vi "Periodic Tasks.vi"(8 "error in":errorcluster) -> ()   [LabVIEW 2018]
doc: "This VI runs in parallel to other tasks. It can contain as many user-defined periodic loops as you need. These can carry out PID or other sorts of timed response."
uses:
  <vilib>/Rock Robotics/WPI/Solenoid/WPI_SolenoidValue.ctl
  <vilib>/Rock Robotics/WPI/Utilities/WPI_GetSetVariantRefNum.vi
  <vilib>/Rock Robotics/WPI/Solenoid/WPI_SolenoidSetEnum.vi
  Robot Global Data.vi
  <vilib>/Rock Robotics/WPI/RobotDrive/WPI_RobotDriveArcadeDrive_Standard(NoSaturation).vi
  <vilib>/Rock Robotics/Network Tables/NT Write Numeric Array.vi
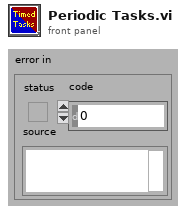
[diagram p1: front panel]
types:
  T1 = typedef "WPI_JoystickDevRef.ctl" = cluster{"Device":T2}
  T2 = typedef "WPI_JoystickDeviceEnum.ctl" = enum16{"USB 0", "USB 1", "USB 2", "USB 3", "USB 4", "USB 5"}
  T3 = typedef "WPI_SolenoidDevRef.ctl" = cluster{"DevStatus":errorcluster, "Pneumatics Control Module":u8, "Forward Solenoid Channel":T4, "Reverse Solenoid Channel":T4}
  T4 = typedef "WPI_SolenoidChannel.ctl" = enum8{"Solenoid 0", "Solenoid 1", "Solenoid 2", "Solenoid 3", "Solenoid 4", "Solenoid 5", "Solenoid 6", "Solenoid 7", "Invalid"}
  T5 = typedef "WPI_AccelerometerDevRef.ctl" = cluster{"DevStatus":errorcluster, "Scaling":T6, "Analog Channels":T7, "I2C Bus":T9, "SPI Bus":T10, "Accel Range":T11, "ADXL Axes":T12, "Handle":i32, "Device Address":u8, "Accel Type":enum16{"Analog", "ADXL345 I2C", "ADXL345 SPI", "Internal", "ADXL362 SPI"}}
  T6 = typedef "WPI_AccelerometerScaling.ctl" = cluster{"Gain (VoltsPerG)":dbl, "Center Voltage":dbl}
  T7 = typedef "WPI_AccelerometerAnalogChannels.ctl" = cluster{"X-Axis":T8, "Y-Axis":T8, "Z-Axis":T8}
  T8 = typedef "FPGA_AIChannel.ctl" = enum8{"AI 0", "AI 1", "AI 2", "AI 3", "AI MXP 0", "AI MXP 1", "AI MXP 2", "AI MXP 3", "Invalid"}
  T9 = typedef "i2c_bus.ctl" = enum16{"I2C On-Board", "I2C MXP", "Invalid"}
  T10 = typedef "spi_bus.ctl" = enum16{"SPI On-Board, CS0", "SPI On-Board, CS1", "SPI On-Board, CS2", "SPI On-Board, CS3", "SPI MXP", "Invalid"}
  T11 = typedef "ADXL345 Range.ctl" = u8
  T12 = typedef "WPI_AccelerometerADXL345 Axes.ctl" = cluster{"X-Axis":bool, "Y-Axis":bool, "Z-Axis":bool}
  T13 = typedef "WPI_SolenoidValue.ctl" = enum16{"Off", "On", "Forward", "Reverse"}
  T14 = typedef "WPI_RobotDriveDevRef.ctl" = cluster{"DevStatus":errorcluster, "Motors[]":T15[], "Square Inputs":bool, "Max Output":dbl}
  T15 = typedef "WPI_MotorControlDeviceRef.ctl" = cluster{"DeviceStatus":errorcluster, "Type":T16, "PWM":cluster{"PWM Channel":T17, "DeadBand":T18}, "CAN":cluster{"Device Number":u8, "SetOutput VI Ref":variant, "GetOutput VI Ref":variant, "Enable VI Ref":variant, "Disable VI Ref":variant, "Data":variant}, "Invert":bool, "DIO PWM":cluster{"PWM \"Enable\" Channel":T17, "DIOChannel":T19, "PWM Rate":dbl}}
  T16 = typedef "WPI_MotorControlType.ctl" = enum16{"PWM", "CAN", "DIO PWM"}
  T17 = typedef "FPGA_DIOPWMChannel.ctl" = enum8{"PWM 0", "PWM 1", "PWM 2", "PWM 3", "PWM 4", "PWM 5", "PWM 6", "PWM 7", "PWM 8", "PWM 9", "PWM MXP 0", "PWM MXP 1", "PWM MXP 2", "PWM MXP 3", "PWM MXP 4", "PWM MXP 5", "PWM MXP 6", "PWM MXP 7", "PWM MXP 8", "PWM MXP 9", "Invalid"}
  T18 = typedef "WPI_PWMDeadband.ctl" = cluster{"Name":string, "maxPositivePwm":i32, "minPositivePwm":i32, "centerPwm":i32, "maxNegativePwm":i32, "minNegativePwm":i32, "angularRange":u16}
  T19 = typedef "FPGA_DIOChannel.ctl" = enum8{"DIO 0", "DIO 1", "DIO 2", "DIO 3", "DIO 4", "DIO 5", "DIO 6", "DIO 7", "DIO 8", "DIO 9", "DIO MXP 0", "DIO MXP 1", "DIO MXP 2", "DIO MXP 3", "DIO MXP 4", "DIO MXP 5", "DIO MXP 6", "DIO MXP 7", "DIO MXP 8", "DIO MXP 9", "DIO MXP 10", "DIO MXP 11", "DIO MXP 12", "DIO MXP 13", "DIO MXP 14", "DIO MXP 15", "SPI Port CS1", "SPI Port CS2", "SPI Port CS3", "SPI Port MISO", "SPI Port MOSI", "Invalid"}
  T20 = cluster{"X-Axis":dbl, "Y-Axis":dbl, "Z-Axis":dbl}
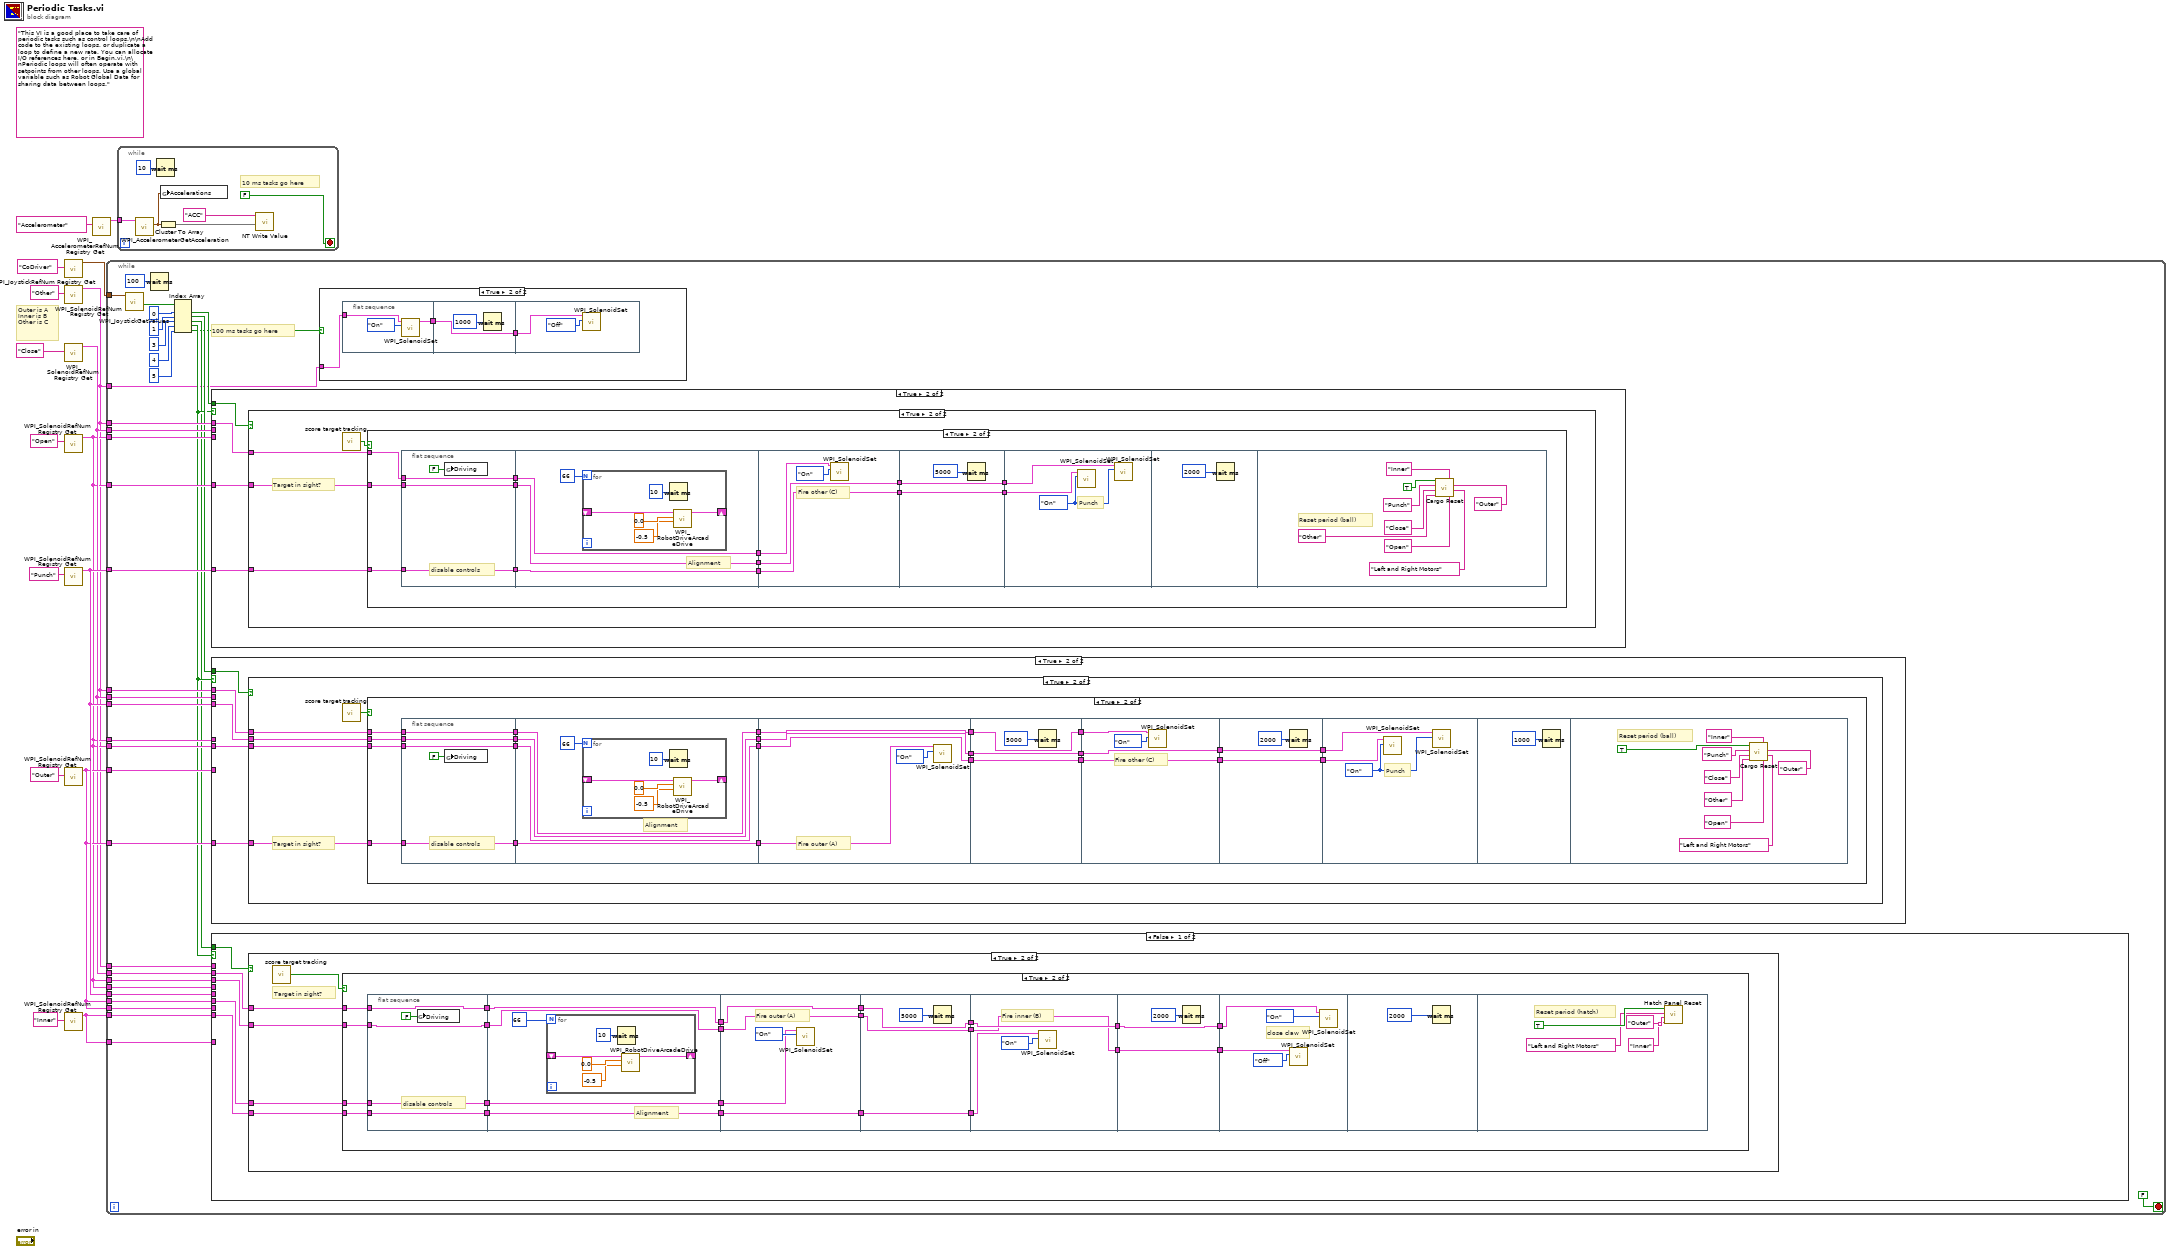
[diagram p0: block diagram]
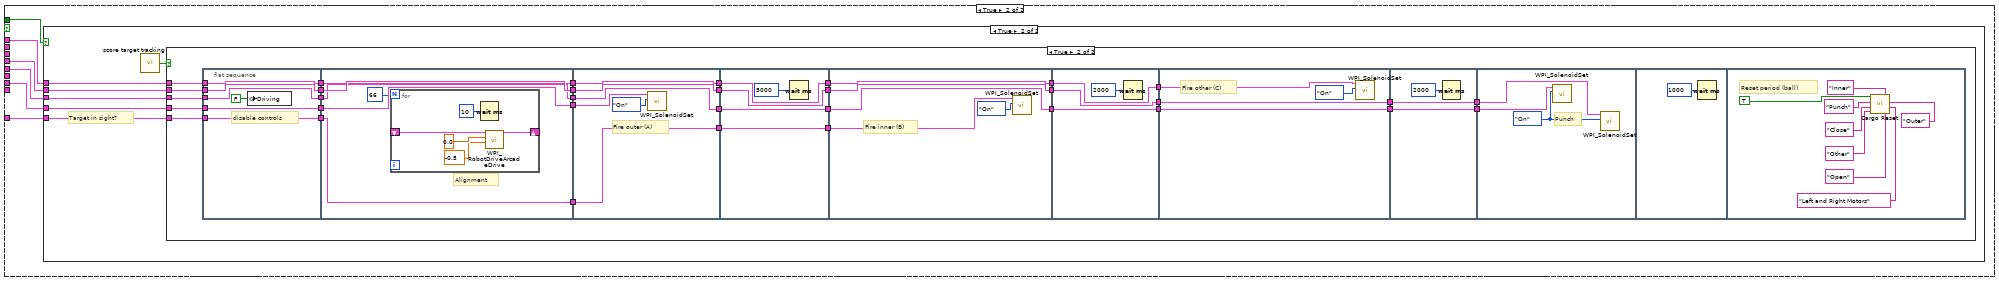
[diagram p5: hidden frame]
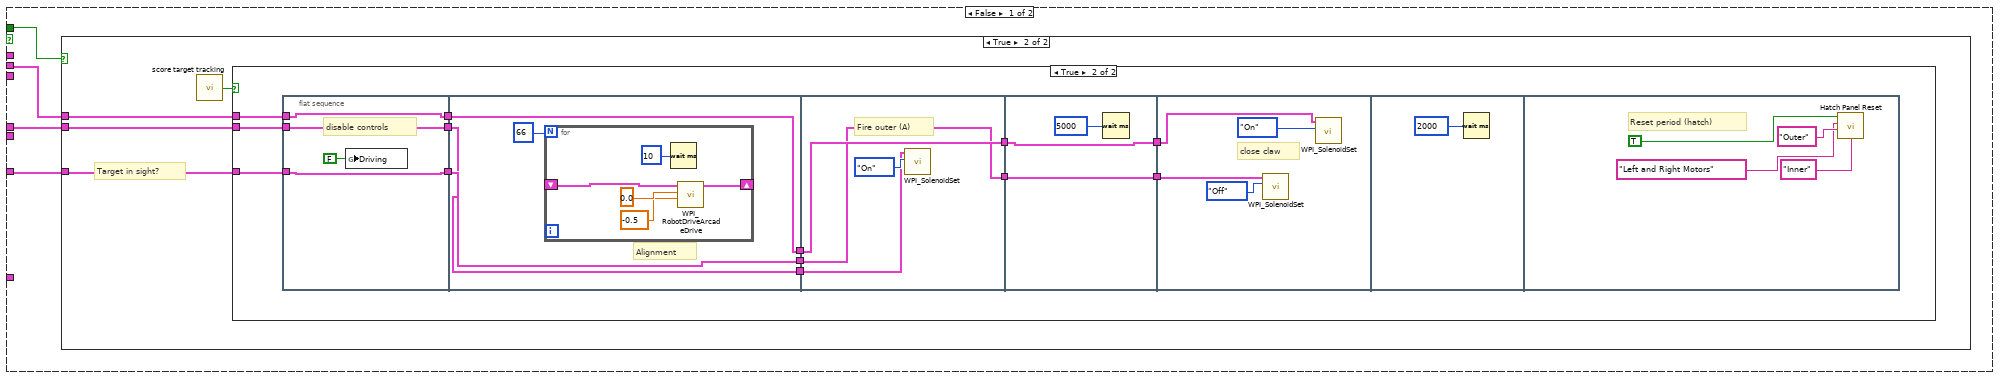
[diagram p8: hidden frame]
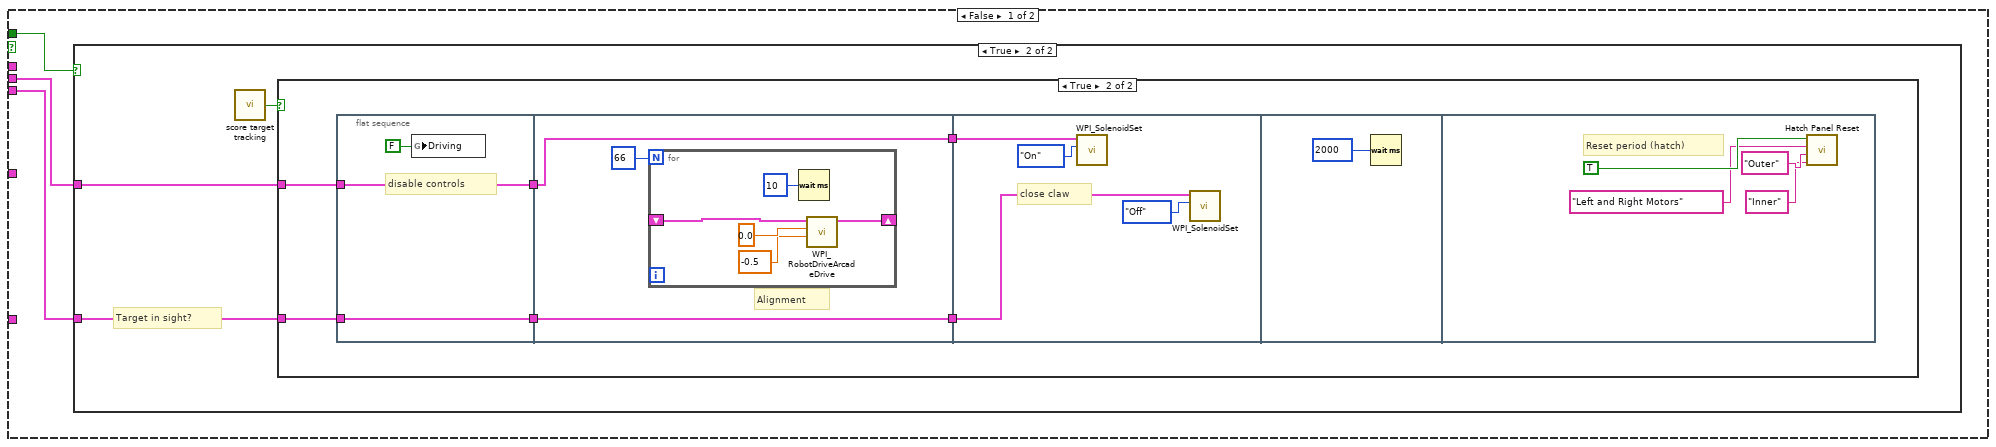
[diagram p13: hidden frame]
diagram:
  (unwired) "This VI is a good place to take care of periodic tasks such as control loops.\n\nAdd code to the existing loops, or duplicate a loop to define a new rate. You can allocate I/O references here, or in Begin.vi.\n\nPeriodic loops will often operate with setpoints from other loops. Use a global variable such as Robot Global Data for sharing data between loops."
  # "Outer is A\nInner is B\nOther is C"
  n1 = call <vilib>:"WPI_JoystickRefNum Registry Get.vi"("refnum name"="CoDriver") -> ("JoystickDevRef"=w12:T1)  [unwired: 9 in, 1 out]
  n2 = call <vilib>:"WPI_SolenoidRefNum Registry Get.vi"("refnum name"="Other") -> ("SolenoidDevRef"=w3:T3)  [unwired: 9 in, 1 out]
  n3 = call <vilib>:"WPI_SolenoidRefNum Registry Get.vi"("refnum name"="Close") -> ("SolenoidDevRef"=w5:T3)  [unwired: 9 in, 1 out]
  n4 = call <vilib>:"WPI_SolenoidRefNum Registry Get.vi"("refnum name"="Open") -> ("SolenoidDevRef"=w4:T3)  [unwired: 9 in, 1 out]
  n5 = call <vilib>:"WPI_SolenoidRefNum Registry Get.vi"("refnum name"="Punch") -> ("SolenoidDevRef"=w8:T3)  [unwired: 9 in, 1 out]
  n6 = call <vilib>:"WPI_SolenoidRefNum Registry Get.vi"("refnum name"="Outer") -> ("SolenoidDevRef"=w7:T3)  [unwired: 9 in, 1 out]
  n7 = call <vilib>:"WPI_SolenoidRefNum Registry Get.vi"("refnum name"="Inner") -> ("SolenoidDevRef"=w6:T3)  [unwired: 9 in, 1 out]
  n8 = call <vilib>:"WPI_AccelerometerRefNum Registry Get.vi"("refnum name"="Accelerometer") -> ("AccelerometerDevRef"=w2:T5)  [unwired: 9 in, 1 out]
  n9 = while {
    tunnel: w12 -> [w50]
    tunnel: w3 -> [w44]
    tunnel: w4 -> [w43]
    tunnel: w8 -> [w42]
    tunnel: w5 -> [w40]
    tunnel: w4 -> [w39]
    tunnel: w8 -> [w38]
    tunnel: w4 -> [w37]
    tunnel: w7 -> [w36]
    tunnel: w3 -> [w35]
    tunnel: w7 -> [w33]
    tunnel: w5 -> [w32]
    tunnel: w4 -> [w31]
    tunnel: w4 -> [w29]
    tunnel: w8 -> [w28]
    tunnel: w7 -> [w27]
    tunnel: w6 -> [w26]
    tunnel: w3 -> [w25]
    tunnel: w7 -> [w24]
    tunnel: w6 -> [w23]
    tunnel: w5 -> [w22]
    tunnel: w4 -> [w21]
    tunnel: w3 -> [w17]
    stop <- FALSE stop-if-true
    # "100 ms tasks go here"
    n10 = call <vilib>:"WPI_JoystickGetValues.vi"("JoystickDevRef"=w50) -> ("Buttons"=w49:bool[])  [unwired: 6 in, 4 out]
    n11 = Wait (ms)(milliseconds to wait=u32 100) -> ()  [unwired: 1 out]
    n12 = Index Array(array=w49, index #1=0, index #2=1, index #3=3, index #4=4, index #5=5) -> (element #1=w41:bool, element #2=w34:bool, element #3=w20:bool, element #4=w30:bool, element #5=w18:bool)
    n13 = case shown="True" w30 {
      tunnel: w44 -> [_ w396]
      tunnel: w43 -> [_ w395]
      tunnel: w42 -> [_ w394]
      tunnel: w41 -> [w363 w393]
      tunnel: w40 -> [w362 _]
      tunnel: w39 -> [w361 _]
      frame False {
        n14 = case shown="True" w363 {
          tunnel: w362 -> [_ w366]
          tunnel: w361 -> [_ w365]
          frame False {
          }
          frame True {
            # "Target in sight?"
            n15 = call "score target tracking.vi"() -> ("Boolean"=w364:bool)
            n16 = case shown="True" w364 {
              tunnel: w366 -> [_ w372]
              tunnel: w365 -> [_ w371]
              frame False {
              }
              frame True {
                n17 = flat-sequence {
                  tunnel: [w375] -> w370
                  tunnel: w372 -> [w375]
                  tunnel: [w374] -> w368
                  tunnel: w371 -> [w374]
                  tunnel: w370 -> [w378]
                  tunnel: [w378] -> w369
                  tunnel: w368 -> [w377]
                  tunnel: [w377] -> w367
                  tunnel: w369 -> [w387]
                  tunnel: w367 -> [w384]
                  frame #0 {
                    # "disable controls"
                    n18 = global write "Robot Global Data.vi" "Driving"(FALSE) -> ()
                  }
                  frame #1 {
                    # "Alignment"
                    n19 = for {
                      N: 66 -> [_]
                      shift-right: [w383] -> _
                      shift-left: _ -> [w382]
                      n20 = Wait (ms)(milliseconds to wait=u32 10) -> ()  [unwired: 1 out]
                      n21 = call-poly <vilib>:"WPI_RobotDriveArcadeDrive.vi"("Y axis value"=-0.5, "X axis value"=0.0, "RobotDriveDevRef"=w382) -> ("RobotDriveDevRef"=w383:T14)  [unwired: 6 in, 2 out]
                    }
                  }
                  frame #2 {
                    # "close claw"
                    n22 = call-poly <vilib>:"WPI_SolenoidSet.vi"("Value"=WPI_SolenoidValue."On", "SolenoidDevRef"=w387) -> ()  [unwired: 8 in, 2 out]
                    n23 = call-poly <vilib>:"WPI_SolenoidSet.vi"("Value"=WPI_SolenoidValue."Off", "SolenoidDevRef"=w384) -> ()  [unwired: 8 in, 2 out]
                  }
                  frame #3 {
                    n24 = Wait (ms)(milliseconds to wait=u32 2000) -> ()  [unwired: 1 out]
                  }
                  frame #4 {
                    # "Reset period (hatch)"
                    n25 = call "Hatch Panel Reset.vi"("InnerRefnum"="Inner", "OuterRefnum"="Outer", "DriveRefnum"="Left and Right Motors", "HatchReset?"=TRUE) -> ()
                  }
                }
              }
            }
          }
        }
      }
      frame True {
        n26 = case shown="True" w393 {
          tunnel: w396 -> [_ w400]
          tunnel: w395 -> [_ w399]
          tunnel: w394 -> [_ w398]
          frame False {
          }
          frame True {
            # "Target in sight?"
            n27 = call "score target tracking.vi"() -> ("Boolean"=w397:bool)
            n28 = case shown="True" w397 {
              tunnel: w400 -> [_ w409]
              tunnel: w399 -> [_ w408]
              tunnel: w398 -> [_ w407]
              frame False {
              }
              frame True {
                n29 = flat-sequence {
                  tunnel: [w417] -> w406
                  tunnel: [w416] -> w404
                  tunnel: [w415] -> w402
                  tunnel: w407 -> [w415]
                  tunnel: w408 -> [w416]
                  tunnel: w409 -> [w417]
                  tunnel: w406 -> [w421]
                  tunnel: [w421] -> w405
                  tunnel: w404 -> [w420]
                  tunnel: [w420] -> w403
                  tunnel: w402 -> [w419]
                  tunnel: [w419] -> w401
                  tunnel: w405 -> [w430]
                  tunnel: [w428] -> w413
                  tunnel: w403 -> [w428]
                  tunnel: [w427] -> w412
                  tunnel: w401 -> [w427]
                  tunnel: w413 -> [w433]
                  tunnel: [w433] -> w411
                  tunnel: w412 -> [w432]
                  tunnel: [w432] -> w410
                  tunnel: w411 -> [w436]
                  tunnel: w410 -> [w435]
                  frame #0 {
                    # "disable controls"
                    n30 = global write "Robot Global Data.vi" "Driving"(FALSE) -> ()
                  }
                  frame #1 {
                    # "Alignment"
                    n31 = for {
                      N: 66 -> [_]
                      shift-right: [w426] -> _
                      shift-left: _ -> [w425]
                      n32 = Wait (ms)(milliseconds to wait=u32 10) -> ()  [unwired: 1 out]
                      n33 = call-poly <vilib>:"WPI_RobotDriveArcadeDrive.vi"("Y axis value"=-0.5, "X axis value"=0.0, "RobotDriveDevRef"=w425) -> ("RobotDriveDevRef"=w426:T14)  [unwired: 6 in, 2 out]
                    }
                  }
                  frame #2 {
                    # "Fire other (C)"
                    n34 = call-poly <vilib>:"WPI_SolenoidSet.vi"("Value"=WPI_SolenoidValue."On", "SolenoidDevRef"=w430) -> ()  [unwired: 8 in, 2 out]
                  }
                  frame #3 {
                    n35 = Wait (ms)(milliseconds to wait=u32 5000) -> ()  [unwired: 1 out]
                  }
                  frame #4 {
                    w434 = WPI_SolenoidValue."On" ("Value")
                    # "Punch"
                    n36 = call-poly <vilib>:"WPI_SolenoidSet.vi"("Value"=w434, "SolenoidDevRef"=w435) -> ()  [unwired: 8 in, 2 out]
                    n37 = call-poly <vilib>:"WPI_SolenoidSet.vi"("Value"=w434, "SolenoidDevRef"=w436) -> ()  [unwired: 8 in, 2 out]
                  }
                  frame #5 {
                    n38 = Wait (ms)(milliseconds to wait=u32 2000) -> ()  [unwired: 1 out]
                  }
                  frame #6 {
                    # "Reset period (ball)"
                    n39 = call "Cargo Reset.vi"("Open Refnum"="Open" ("refnum name"), "Drive Refnum"="Left and Right Motors" ("DriveRefnum"), "Outer Refnum"="Outer" ("OuterRefnum"), "Inner Refnum"="Inner" ("InnerRefnum"), "Other Refnum"="Other" ("refnum name"), "Close Refnum"="Close" ("refnum name"), "Punch Refnum"="Punch" ("refnum name"), "Ball reset?"=TRUE) -> ()
                  }
                }
              }
            }
          }
        }
      }
    }
    n40 = case shown="True" w30 {
      tunnel: w38 -> [_ w290]
      tunnel: w37 -> [_ w289]
      tunnel: w36 -> [_ w288]
      tunnel: w35 -> [_ w287]
      tunnel: w34 -> [w239 w286]
      tunnel: w33 -> [w238 _]
      tunnel: w32 -> [w237 _]
      tunnel: w31 -> [w236 _]
      frame False {
        n41 = case shown="True" w239 {
          tunnel: w238 -> [_ w243]
          tunnel: w237 -> [_ w242]
          tunnel: w236 -> [_ w241]
          frame False {
          }
          frame True {
            # "Target in sight?"
            n42 = call "score target tracking.vi"() -> ("Boolean"=w240:bool)
            n43 = case shown="True" w240 {
              tunnel: w243 -> [_ w252]
              tunnel: w242 -> [_ w251]
              tunnel: w241 -> [_ w250]
              frame False {
              }
              frame True {
                n44 = flat-sequence {
                  tunnel: [w260] -> w249
                  tunnel: w252 -> [w260]
                  tunnel: [w259] -> w247
                  tunnel: w251 -> [w259]
                  tunnel: [w258] -> w245
                  tunnel: w250 -> [w258]
                  tunnel: w249 -> [w264]
                  tunnel: [w264] -> w248
                  tunnel: w247 -> [w263]
                  tunnel: [w263] -> w246
                  tunnel: w245 -> [w262]
                  tunnel: [w262] -> w244
                  tunnel: w248 -> [w272]
                  tunnel: [w271] -> w256
                  tunnel: w246 -> [w271]
                  tunnel: [w270] -> w255
                  tunnel: w244 -> [w270]
                  tunnel: w256 -> [w276]
                  tunnel: [w276] -> w254
                  tunnel: w255 -> [w275]
                  tunnel: [w275] -> w253
                  tunnel: w254 -> [w280]
                  tunnel: w253 -> [w277]
                  frame #0 {
                    # "disable controls"
                    n45 = global write "Robot Global Data.vi" "Driving"(FALSE) -> ()
                  }
                  frame #1 {
                    # "Alignment"
                    n46 = for {
                      N: 66 -> [_]
                      shift-right: [w269] -> _
                      shift-left: _ -> [w268]
                      n47 = Wait (ms)(milliseconds to wait=u32 10) -> ()  [unwired: 1 out]
                      n48 = call-poly <vilib>:"WPI_RobotDriveArcadeDrive.vi"("Y axis value"=-0.5, "X axis value"=0.0, "RobotDriveDevRef"=w268) -> ("RobotDriveDevRef"=w269:T14)  [unwired: 6 in, 2 out]
                    }
                  }
                  frame #2 {
                    # "Fire outer (A)"
                    n49 = call-poly <vilib>:"WPI_SolenoidSet.vi"("Value"=WPI_SolenoidValue."On", "SolenoidDevRef"=w272) -> ()  [unwired: 8 in, 2 out]
                  }
                  frame #3 {
                    n50 = Wait (ms)(milliseconds to wait=u32 5000) -> ()  [unwired: 1 out]
                  }
                  frame #4 {
                    # "close claw"
                    n51 = call-poly <vilib>:"WPI_SolenoidSet.vi"("Value"=WPI_SolenoidValue."Off", "SolenoidDevRef"=w277) -> ()  [unwired: 8 in, 2 out]
                    n52 = call-poly <vilib>:"WPI_SolenoidSet.vi"("Value"=WPI_SolenoidValue."On", "SolenoidDevRef"=w280) -> ()  [unwired: 8 in, 2 out]
                  }
                  frame #5 {
                    n53 = Wait (ms)(milliseconds to wait=u32 2000) -> ()  [unwired: 1 out]
                  }
                  frame #6 {
                    # "Reset period (hatch)"
                    n54 = call "Hatch Panel Reset.vi"("InnerRefnum"="Inner", "OuterRefnum"="Outer", "DriveRefnum"="Left and Right Motors", "HatchReset?"=TRUE) -> ()
                  }
                }
              }
            }
          }
        }
      }
      frame True {
        n55 = case shown="True" w286 {
          tunnel: w290 -> [_ w295]
          tunnel: w289 -> [_ w294]
          tunnel: w288 -> [_ w293]
          tunnel: w287 -> [_ w292]
          frame False {
          }
          frame True {
            # "Target in sight?"
            n56 = call "score target tracking.vi"() -> ("Boolean"=w291:bool)
            n57 = case shown="True" w291 {
              tunnel: w295 -> [_ w307]
              tunnel: w294 -> [_ w306]
              tunnel: w293 -> [_ w305]
              tunnel: w292 -> [_ w304]
              frame False {
              }
              frame True {
                n58 = flat-sequence {
                  tunnel: [w322] -> w303
                  tunnel: w307 -> [w322]
                  tunnel: [w321] -> w301
                  tunnel: w306 -> [w321]
                  tunnel: [w320] -> w299
                  tunnel: w305 -> [w320]
                  tunnel: [w319] -> w297
                  tunnel: w304 -> [w319]
                  tunnel: w303 -> [w327]
                  tunnel: [w327] -> w302
                  tunnel: w301 -> [w326]
                  tunnel: [w326] -> w300
                  tunnel: w299 -> [w325]
                  tunnel: [w325] -> w298
                  tunnel: w297 -> [w324]
                  tunnel: [w324] -> w296
                  tunnel: [w337] -> w317
                  tunnel: w302 -> [w337]
                  tunnel: [w336] -> w316
                  tunnel: w300 -> [w336]
                  tunnel: w298 -> [w334]
                  tunnel: [w333] -> w315
                  tunnel: w296 -> [w333]
                  tunnel: w317 -> [w341]
                  tunnel: [w341] -> w314
                  tunnel: w316 -> [w340]
                  tunnel: [w340] -> w313
                  tunnel: w315 -> [w339]
                  tunnel: [w339] -> w312
                  tunnel: [w345] -> w311
                  tunnel: w314 -> [w345]
                  tunnel: [w344] -> w310
                  tunnel: w313 -> [w344]
                  tunnel: w312 -> [w342]
                  tunnel: w311 -> [w348]
                  tunnel: [w348] -> w309
                  tunnel: w310 -> [w347]
                  tunnel: [w347] -> w308
                  tunnel: w309 -> [w351]
                  tunnel: w308 -> [w350]
                  frame #0 {
                    # "disable controls"
                    n59 = global write "Robot Global Data.vi" "Driving"(FALSE) -> ()
                  }
                  frame #1 {
                    # "Alignment"
                    n60 = for {
                      N: 66 -> [_]
                      shift-right: [w332] -> _
                      shift-left: _ -> [w331]
                      n61 = Wait (ms)(milliseconds to wait=u32 10) -> ()  [unwired: 1 out]
                      n62 = call-poly <vilib>:"WPI_RobotDriveArcadeDrive.vi"("Y axis value"=-0.5, "X axis value"=0.0, "RobotDriveDevRef"=w331) -> ("RobotDriveDevRef"=w332:T14)  [unwired: 6 in, 2 out]
                    }
                  }
                  frame #2 {
                    # "Fire outer (A)"
                    n63 = call-poly <vilib>:"WPI_SolenoidSet.vi"("Value"=WPI_SolenoidValue."On", "SolenoidDevRef"=w334) -> ()  [unwired: 8 in, 2 out]
                  }
                  frame #3 {
                    n64 = Wait (ms)(milliseconds to wait=u32 5000) -> ()  [unwired: 1 out]
                  }
                  frame #4 {
                    # "Fire other (C)"
                    n65 = call-poly <vilib>:"WPI_SolenoidSet.vi"("Value"=WPI_SolenoidValue."On", "SolenoidDevRef"=w342) -> ()  [unwired: 8 in, 2 out]
                  }
                  frame #5 {
                    n66 = Wait (ms)(milliseconds to wait=u32 2000) -> ()  [unwired: 1 out]
                  }
                  frame #6 {
                    w349 = WPI_SolenoidValue."On" ("Value")
                    # "Punch"
                    n67 = call-poly <vilib>:"WPI_SolenoidSet.vi"("Value"=w349, "SolenoidDevRef"=w350) -> ()  [unwired: 8 in, 2 out]
                    n68 = call-poly <vilib>:"WPI_SolenoidSet.vi"("Value"=w349, "SolenoidDevRef"=w351) -> ()  [unwired: 8 in, 2 out]
                  }
                  frame #7 {
                    n69 = Wait (ms)(milliseconds to wait=u32 1000) -> ()  [unwired: 1 out]
                  }
                  frame #8 {
                    # "Reset period (ball)"
                    n70 = call "Cargo Reset.vi"("Open Refnum"="Open" ("refnum name"), "Drive Refnum"="Left and Right Motors" ("DriveRefnum"), "Outer Refnum"="Outer" ("OuterRefnum"), "Inner Refnum"="Inner" ("InnerRefnum"), "Other Refnum"="Other" ("refnum name"), "Close Refnum"="Close" ("refnum name"), "Punch Refnum"="Punch" ("refnum name"), "Ball reset?"=TRUE) -> ()
                  }
                }
              }
            }
          }
        }
      }
    }
    n71 = case shown="False" w30 {
      tunnel: w29 -> [_ w140]
      tunnel: w28 -> [_ w139]
      tunnel: w27 -> [_ w138]
      tunnel: w26 -> [_ w137]
      tunnel: w25 -> [_ w136]
      tunnel: w24 -> [w67 _]
      tunnel: w23 -> [w66 _]
      tunnel: w22 -> [w65 _]
      tunnel: w21 -> [w64 _]
      tunnel: w20 -> [w63 w135]
      frame False {
        n72 = case shown="True" w63 {
          tunnel: w67 -> [_ w72]
          tunnel: w66 -> [_ w71]
          tunnel: w65 -> [_ w70]
          tunnel: w64 -> [_ w69]
          frame False {
          }
          frame True {
            # "Target in sight?"
            n73 = call "score target tracking.vi"() -> ("Boolean"=w68:bool)
            n74 = case shown="True" w68 {
              tunnel: w72 -> [_ w84]
              tunnel: w71 -> [_ w83]
              tunnel: w70 -> [_ w82]
              tunnel: w69 -> [_ w81]
              frame False {
              }
              frame True {
                n75 = flat-sequence {
                  tunnel: [w99] -> w80
                  tunnel: w84 -> [w99]
                  tunnel: [w98] -> w78
                  tunnel: w83 -> [w98]
                  tunnel: [w97] -> w76
                  tunnel: w82 -> [w97]
                  tunnel: [w96] -> w74
                  tunnel: w81 -> [w96]
                  tunnel: w80 -> [w104]
                  tunnel: [w104] -> w79
                  tunnel: w78 -> [w103]
                  tunnel: [w103] -> w77
                  tunnel: w76 -> [w102]
                  tunnel: [w102] -> w75
                  tunnel: w74 -> [w101]
                  tunnel: [w101] -> w73
                  tunnel: w79 -> [w113]
                  tunnel: [w112] -> w94
                  tunnel: w77 -> [w112]
                  tunnel: [w111] -> w93
                  tunnel: w75 -> [w111]
                  tunnel: [w110] -> w92
                  tunnel: w73 -> [w110]
                  tunnel: w94 -> [w118]
                  tunnel: [w118] -> w91
                  tunnel: w93 -> [w117]
                  tunnel: [w117] -> w90
                  tunnel: w92 -> [w116]
                  tunnel: [w116] -> w89
                  tunnel: w91 -> [w121]
                  tunnel: [w120] -> w88
                  tunnel: w90 -> [w120]
                  tunnel: [w119] -> w87
                  tunnel: w89 -> [w119]
                  tunnel: w88 -> [w125]
                  tunnel: [w125] -> w86
                  tunnel: w87 -> [w124]
                  tunnel: [w124] -> w85
                  tunnel: w86 -> [w127]
                  tunnel: w85 -> [w126]
                  frame #0 {
                    # "disable controls"
                    n76 = global write "Robot Global Data.vi" "Driving"(FALSE) -> ()
                  }
                  frame #1 {
                    # "Alignment"
                    n77 = for {
                      N: 66 -> [_]
                      shift-right: [w109] -> _
                      shift-left: _ -> [w108]
                      n78 = Wait (ms)(milliseconds to wait=u32 10) -> ()  [unwired: 1 out]
                      n79 = call-poly <vilib>:"WPI_RobotDriveArcadeDrive.vi"("Y axis value"=-0.5, "X axis value"=0.0, "RobotDriveDevRef"=w108) -> ("RobotDriveDevRef"=w109:T14)  [unwired: 6 in, 2 out]
                    }
                  }
                  frame #2 {
                    # "Fire outer (A)"
                    n80 = call-poly <vilib>:"WPI_SolenoidSet.vi"("Value"=WPI_SolenoidValue."On", "SolenoidDevRef"=w113) -> ()  [unwired: 8 in, 2 out]
                  }
                  frame #3 {
                    n81 = Wait (ms)(milliseconds to wait=u32 5000) -> ()  [unwired: 1 out]
                  }
                  frame #4 {
                    # "Fire inner (B)"
                    n82 = call-poly <vilib>:"WPI_SolenoidSet.vi"("Value"=WPI_SolenoidValue."On", "SolenoidDevRef"=w121) -> ()  [unwired: 8 in, 2 out]
                  }
                  frame #5 {
                    n83 = Wait (ms)(milliseconds to wait=u32 2000) -> ()  [unwired: 1 out]
                  }
                  frame #6 {
                    # "close claw"
                    n84 = call-poly <vilib>:"WPI_SolenoidSet.vi"("Value"=WPI_SolenoidValue."Off", "SolenoidDevRef"=w126) -> ()  [unwired: 8 in, 2 out]
                    n85 = call-poly <vilib>:"WPI_SolenoidSet.vi"("Value"=WPI_SolenoidValue."On", "SolenoidDevRef"=w127) -> ()  [unwired: 8 in, 2 out]
                  }
                  frame #7 {
                    n86 = Wait (ms)(milliseconds to wait=u32 2000) -> ()  [unwired: 1 out]
                  }
                  frame #8 {
                    # "Reset period (hatch)"
                    n87 = call "Hatch Panel Reset.vi"("InnerRefnum"="Inner", "OuterRefnum"="Outer", "DriveRefnum"="Left and Right Motors", "HatchReset?"=TRUE) -> ()
                  }
                }
              }
            }
          }
        }
      }
      frame True {
        n88 = case shown="True" w135 {
          tunnel: w140 -> [_ w146]
          tunnel: w139 -> [_ w145]
          tunnel: w138 -> [_ w144]
          tunnel: w137 -> [_ w143]
          tunnel: w136 -> [_ w142]
          frame False {
          }
          frame True {
            # "Target in sight?"
            n89 = call "score target tracking.vi"() -> ("Boolean"=w141:bool)
            n90 = case shown="True" w141 {
              tunnel: w146 -> [_ w161]
              tunnel: w145 -> [_ w160]
              tunnel: w144 -> [_ w159]
              tunnel: w143 -> [_ w158]
              tunnel: w142 -> [_ w157]
              frame False {
              }
              frame True {
                n91 = flat-sequence {
                  tunnel: [w185] -> w156
                  tunnel: w161 -> [w185]
                  tunnel: [w184] -> w154
                  tunnel: w160 -> [w184]
                  tunnel: [w183] -> w152
                  tunnel: w159 -> [w183]
                  tunnel: [w182] -> w150
                  tunnel: w158 -> [w182]
                  tunnel: [w181] -> w148
                  tunnel: w157 -> [w181]
                  tunnel: w156 -> [w191]
                  tunnel: [w191] -> w155
                  tunnel: w154 -> [w190]
                  tunnel: [w190] -> w153
                  tunnel: w152 -> [w189]
                  tunnel: [w189] -> w151
                  tunnel: w150 -> [w188]
                  tunnel: [w188] -> w149
                  tunnel: w148 -> [w187]
                  tunnel: [w187] -> w147
                  tunnel: [w202] -> w179
                  tunnel: w155 -> [w202]
                  tunnel: [w201] -> w178
                  tunnel: w153 -> [w201]
                  tunnel: w151 -> [w199]
                  tunnel: [w198] -> w177
                  tunnel: w149 -> [w198]
                  tunnel: [w197] -> w176
                  tunnel: w147 -> [w197]
                  tunnel: w179 -> [w207]
                  tunnel: [w207] -> w175
                  tunnel: w178 -> [w206]
                  tunnel: [w206] -> w174
                  tunnel: w177 -> [w205]
                  tunnel: [w205] -> w173
                  tunnel: w176 -> [w204]
                  tunnel: [w204] -> w172
                  tunnel: [w212] -> w171
                  tunnel: w175 -> [w212]
                  tunnel: [w211] -> w170
                  tunnel: w174 -> [w211]
                  tunnel: w173 -> [w209]
                  tunnel: [w208] -> w169
                  tunnel: w172 -> [w208]
                  tunnel: w171 -> [w216]
                  tunnel: [w216] -> w168
                  tunnel: w170 -> [w215]
                  tunnel: [w215] -> w167
                  tunnel: w169 -> [w214]
                  tunnel: [w214] -> w166
                  tunnel: [w220] -> w165
                  tunnel: w168 -> [w220]
                  tunnel: [w219] -> w164
                  tunnel: w167 -> [w219]
                  tunnel: w166 -> [w217]
                  tunnel: w165 -> [w223]
                  tunnel: [w223] -> w163
                  tunnel: w164 -> [w222]
                  tunnel: [w222] -> w162
                  tunnel: w163 -> [w225]
                  tunnel: w162 -> [w224]
                  frame #0 {
                    # "disable controls"
                    n92 = global write "Robot Global Data.vi" "Driving"(FALSE) -> ()
                  }
                  frame #1 {
                    # "Alignment"
                    n93 = for {
                      N: 66 -> [_]
                      shift-right: [w196] -> _
                      shift-left: _ -> [w195]
                      n94 = Wait (ms)(milliseconds to wait=u32 10) -> ()  [unwired: 1 out]
                      n95 = call-poly <vilib>:"WPI_RobotDriveArcadeDrive.vi"("Y axis value"=-0.5, "X axis value"=0.0, "RobotDriveDevRef"=w195) -> ("RobotDriveDevRef"=w196:T14)  [unwired: 6 in, 2 out]
                    }
                  }
                  frame #2 {
                    # "Fire outer (A)"
                    n96 = call-poly <vilib>:"WPI_SolenoidSet.vi"("Value"=WPI_SolenoidValue."On", "SolenoidDevRef"=w199) -> ()  [unwired: 8 in, 2 out]
                  }
                  frame #3 {
                    n97 = Wait (ms)(milliseconds to wait=u32 5000) -> ()  [unwired: 1 out]
                  }
                  frame #4 {
                    # "Fire inner (B)"
                    n98 = call-poly <vilib>:"WPI_SolenoidSet.vi"("Value"=WPI_SolenoidValue."On", "SolenoidDevRef"=w209) -> ()  [unwired: 8 in, 2 out]
                  }
                  frame #5 {
                    n99 = Wait (ms)(milliseconds to wait=u32 2000) -> ()  [unwired: 1 out]
                  }
                  frame #6 {
                    # "Fire other (C)"
                    n100 = call-poly <vilib>:"WPI_SolenoidSet.vi"("Value"=WPI_SolenoidValue."On", "SolenoidDevRef"=w217) -> ()  [unwired: 8 in, 2 out]
                  }
                  frame #7 {
                    n101 = Wait (ms)(milliseconds to wait=u32 2000) -> ()  [unwired: 1 out]
                  }
                  frame #8 {
                    w226 = WPI_SolenoidValue."On" ("Value")
                    # "Punch"
                    n102 = call-poly <vilib>:"WPI_SolenoidSet.vi"("Value"=w226, "SolenoidDevRef"=w224) -> ()  [unwired: 8 in, 2 out]
                    n103 = call-poly <vilib>:"WPI_SolenoidSet.vi"("Value"=w226, "SolenoidDevRef"=w225) -> ()  [unwired: 8 in, 2 out]
                  }
                  frame #9 {
                    n104 = Wait (ms)(milliseconds to wait=u32 1000) -> ()  [unwired: 1 out]
                  }
                  frame #10 {
                    # "Reset period (ball)"
                    n105 = call "Cargo Reset.vi"("Open Refnum"="Open" ("refnum name"), "Drive Refnum"="Left and Right Motors" ("DriveRefnum"), "Outer Refnum"="Outer" ("OuterRefnum"), "Inner Refnum"="Inner" ("InnerRefnum"), "Other Refnum"="Other" ("refnum name"), "Close Refnum"="Close" ("refnum name"), "Punch Refnum"="Punch" ("refnum name"), "Ball reset?"=TRUE) -> ()
                  }
                }
              }
            }
          }
        }
      }
    }
    n106 = case shown="True" w18 {
      tunnel: w17 -> [_ w55]
      frame False {
      }
      frame True {
        n107 = flat-sequence {
          tunnel: w55 -> [w58]
          tunnel: [w57] -> w53
          tunnel: [w60] -> w54
          tunnel: w53 -> [w60]
          tunnel: w54 -> [w62]
          frame #0 {
            n108 = call-poly <vilib>:"WPI_SolenoidSet.vi"("Value"=WPI_SolenoidValue."On", "SolenoidDevRef"=w58) -> ("SolenoidDevRef"=w57:T3)  [unwired: 8 in, 1 out]
          }
          frame #1 {
            n109 = Wait (ms)(milliseconds to wait=u32 1000) -> ()  [unwired: 1 out]
          }
          frame #2 {
            n110 = call-poly <vilib>:"WPI_SolenoidSet.vi"("Value"=WPI_SolenoidValue."Off", "SolenoidDevRef"=w62) -> ()  [unwired: 8 in, 2 out]
          }
        }
      }
    }
  }
  n111 = while {
    tunnel: w2 -> [w450]
    stop <- FALSE stop-if-true
    # "10 ms tasks go here"
    n112 = call <vilib>:"WPI_AccelerometerGetAcceleration.vi"("AccelerometerDevRef"=w450) -> ("Accelerations"=w446:T20)  [unwired: 8 in, 2 out]
    n113 = Wait (ms)(milliseconds to wait=u32 10) -> ()  [unwired: 1 out]
    n114 = Cluster To Array(cluster=w446) -> (array=w449:dbl[])
    n115 = global write "Robot Global Data.vi" "Accelerations"(w446) -> ()
    n116 = call-poly <vilib>:"NT Write Value.vi"("Numeric Array"=w449, "Name"="ACC") -> ()  [unwired: 9 in, 1 out]
  }
